vi "PhotonPoseEstimator_closestToCameraHeightStrategy.vi"(10 "CameraResult":T11, 11 "PhotonPoseEstimator_REF":T1) -> (1 "Pos Found":bool, 3 "PhotonEstimatedRobotPose":T2={"EstimatedPose"={"Translation3d"={"X"=0.0, "Y"=0.0, "Z"=0.0}, "Rotation3d"={"Q_quaternion"={"R"=1.0, "V"=[0.0, 0.0, 0.0]}}}, "TimeStamp_Seconds"=0.0, "targetsUsed"=[], "Strategy"=enum."LOWEST_AMBIGUITY"} {"targetsUsed"."AltCameraToTarget"."TRANSLATION3D"."Z" format="%14.3f"; "targetsUsed"."AltCameraToTarget"."TRANSLATION3D"."Y" format="%14.3f"; "targetsUsed"."AltCameraToTarget"."TRANSLATION3D"."X" format="%14.3f"; "targetsUsed"."BestCameraToTarget"."TRANSLATION3D"."Z" format="%14.3f"; "targetsUsed"."BestCameraToTarget"."TRANSLATION3D"."Y" format="%14.3f"; "targetsUsed"."BestCameraToTarget"."TRANSLATION3D"."X" format="%14.3f"; "EstimatedPose"."Translation3d"."Z" format="%14.3f"; "EstimatedPose"."Translation3d"."Y" format="%14.3f"; "EstimatedPose"."Translation3d"."X" format="%14.3f"})   [LabVIEW 2019, in "PhotonVisionLib.lvlib"]
doc: "This is an internal function. Use Update or Update_Pipeline instead of this function.\n\nDetermine the best target based on the target height closed to the camera height."
uses:
  PhotonVisionLib.lvlib
  <vilib>/Rock Robotics/WPI/ThirdParty/JAS_Junk/TrajLib/TypeDef/QUATERNION.ctl
  <vilib>/Rock Robotics/WPI/ThirdParty/JAS_Junk/TrajLib/Trajectory_Library.lvlib
  <vilib>/Rock Robotics/WPI/ThirdParty/JAS_Junk/TrajLib/TypeDef/ROTATION3D.ctl
  <vilib>/Rock Robotics/WPI/ThirdParty/JAS_Junk/TrajLib/TypeDef/TRANSLATION3D.ctl
  <vilib>/Rock Robotics/WPI/ThirdParty/JAS_Junk/TrajLib/TypeDef/POSE3D.ctl
  TypeDef/PhotonEstimatedRobotPoseType.ctl
  Enum/PhotonPoseStrategy_ENUM.ctl
  TypeDef/TargetCornerType.ctl
  <vilib>/Rock Robotics/WPI/ThirdParty/JAS_Junk/TrajLib/TypeDef/TRANSFORM3D.ctl
  TypeDef/PhotonTrackedTargetType.ctl
  TypeDef/PhotonPipelineResultType.ctl
  <vilib>/Rock Robotics/WPI/ThirdParty/JAS_Junk/TrajLib/TypeDef/AprilTag.ctl
  <vilib>/Rock Robotics/WPI/ThirdParty/JAS_Junk/TrajLib/Enum/AprilTagFieldLayoutOrignPosition_ENUM.ctl
  <vilib>/Rock Robotics/WPI/ThirdParty/JAS_Junk/TrajLib/TypeDef/AprilTagFieldLayout.ctl
  TypeDef/PhotonPoseEstimatorType.ctl
  TypeDef/PhotonPNPResultType.ctl
  TypeDef/PhotonMultiTargetPNPResultType.ctl
  TypeDef/PhotonTargetModel.ctl
  Ref/PhotonPipelineResult_REF.ctl
  Ref/PhotonPoseEstimator_REF.ctl
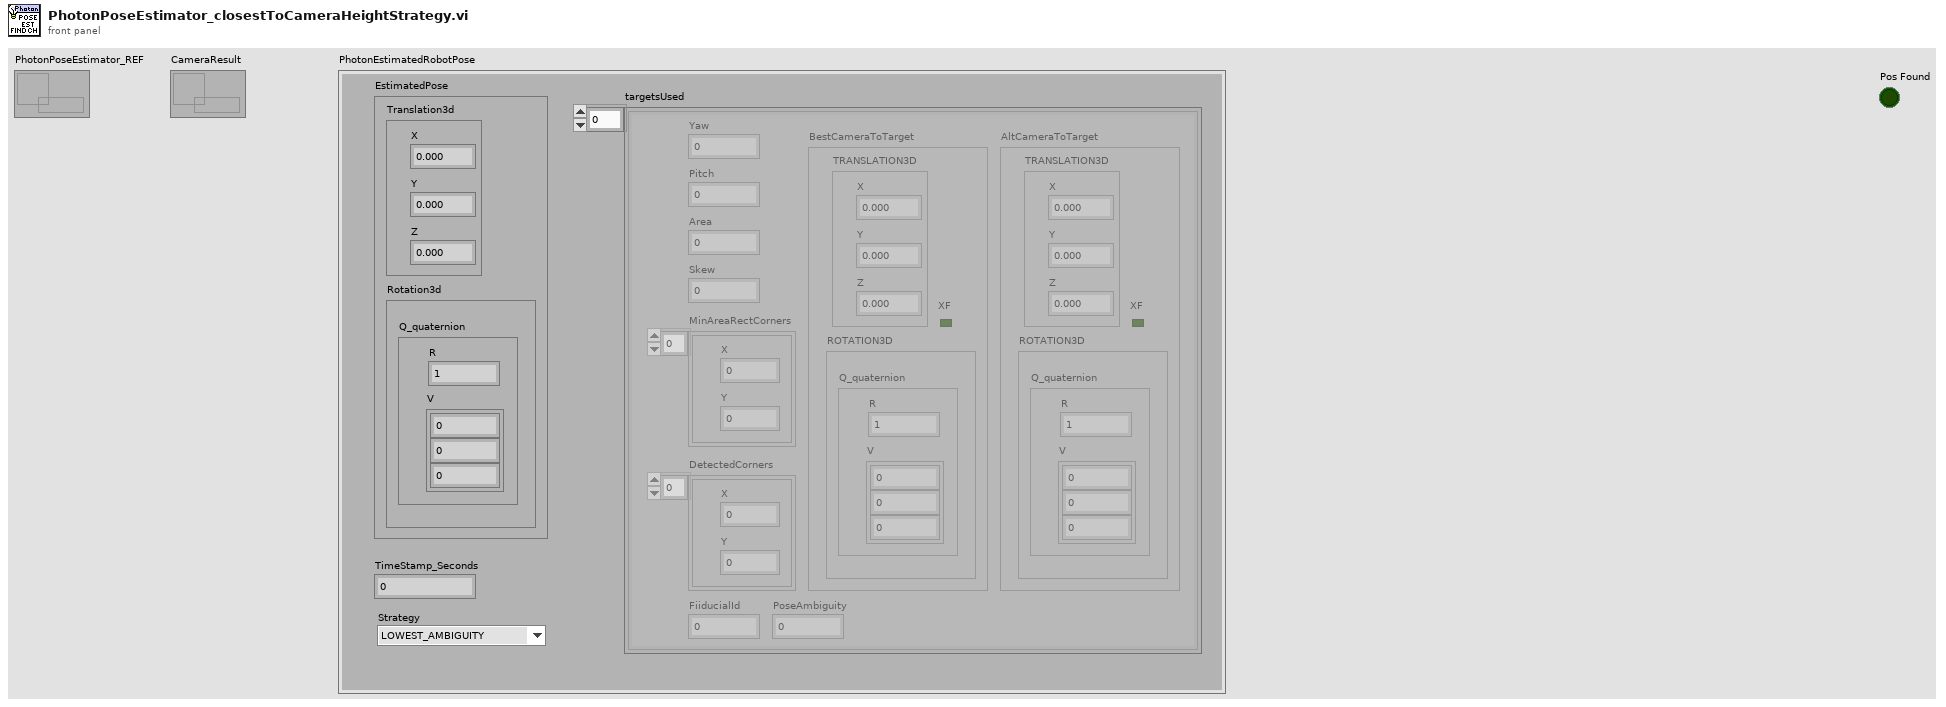
[diagram p1: front panel]
types:
  T1 = typedef "PhotonVisionLib.lvlib/PhotonPoseEstimator_REF.ctl" = refnum<data-value>
  T2 = typedef "PhotonVisionLib.lvlib/PhotonEstimatedRobotPoseType.ctl" = cluster{"EstimatedPose":T3, "TimeStamp_Seconds":dbl, "targetsUsed":T7[], "Strategy":T10}
  T3 = typedef "Trajectory_Library.lvlib/POSE3D.ctl" = cluster{"Translation3d":T4, "Rotation3d":T5}
  T4 = typedef "Trajectory_Library.lvlib/TRANSLATION3D.ctl" = cluster{"X":dbl, "Y":dbl, "Z":dbl}
  T5 = typedef "Trajectory_Library.lvlib/ROTATION3D.ctl" = cluster{"Q_quaternion":T6}
  T6 = typedef "Trajectory_Library.lvlib/QUATERNION.ctl" = cluster{"R":dbl, "V":dbl[]}
  T7 = typedef "PhotonVisionLib.lvlib/PhotonTrackedTargetType.ctl" = cluster{"Yaw":dbl, "Pitch":dbl, "Area":dbl, "Skew":dbl, "MinAreaRectCorners":T8[], "BestCameraToTarget":T9, "FiiducialId":i32, "AltCameraToTarget":T9, "PoseAmbiguity":dbl, "DetectedCorners":T8[]}
  T8 = typedef "PhotonVisionLib.lvlib/TargetCornerType.ctl" = cluster{"X":dbl, "Y":dbl}
  T9 = typedef "Trajectory_Library.lvlib/TRANSFORM3D.ctl" = cluster{"TRANSLATION3D":T4, "ROTATION3D":T5, "XF":bool}
  T10 = typedef "PhotonVisionLib.lvlib/PhotonPoseStrategy_ENUM.ctl" = enum16{"LOWEST_AMBIGUITY", "CLOSEST_TO_CAMERA_HEIGHT", "CLOSEST_TO_REFERENCE_POSE", "CLOSEST_TO_LAST_POSE", "AVERAGE_BEST_TARGETS", "MULTI_TAG_PNP_ON_COPROCESSOR", "MULTI_TAG_PNP_ON_RIO"}
  T11 = typedef "PhotonVisionLib.lvlib/PhotonPipelineResult_REF.ctl" = refnum<data-value>
  T12 = typedef "Trajectory_Library.lvlib/AprilTagFieldLayout.ctl" = cluster{"AprilTagMap":map{i32, T13}, "FieldLength":dbl, "FieldWidth":dbl, "OriginPosition ":T14, "OriginPose3d":T3}
  T13 = typedef "Trajectory_Library.lvlib/AprilTag.ctl" = cluster{"ID":i32, "POSE3D":T3}
  T14 = typedef "Trajectory_Library.lvlib/AprilTagFieldLayoutOrignPosition_ENUM.ctl" = enum16{"kBlueAllianceWallRightSide,", "kRedAllianceWallRightSide,"}
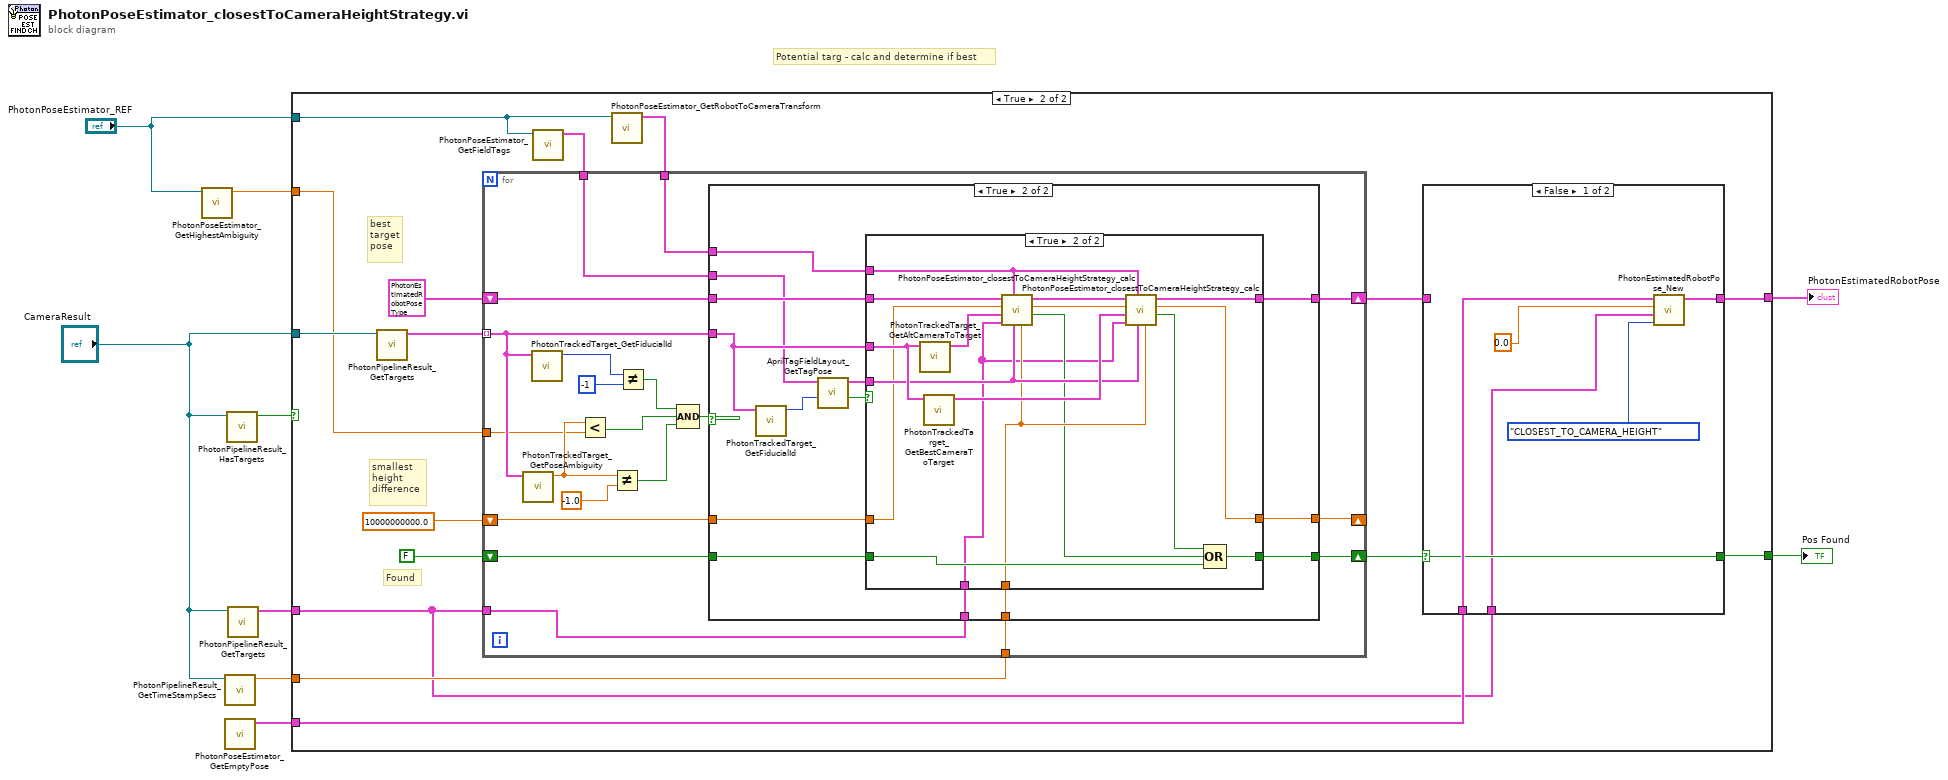
[diagram p0: block diagram]
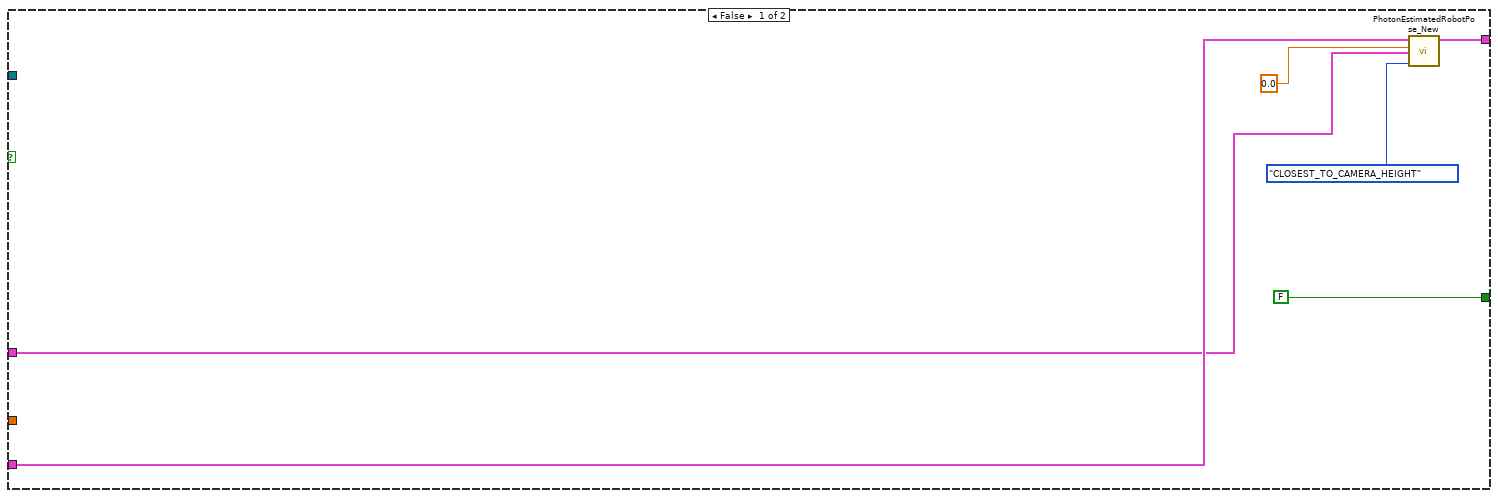
[diagram p2: hidden frame]
diagram:
  # "Potential targ - calc and determine if best"
  n1 = call "PhotonPoseEstimator_GetHighestAmbiguity.vi"("PhotonPoseEstimator"="PhotonPoseEstimator_REF") -> ("HighestAmbiguity"=w3:dbl)  [unwired: 10 in]
  n2 = call "PhotonPipelineResult_GetTimeStampSecs.vi"("PhotonPipelineResult_REF"="CameraResult") -> ("TimeStampSec"=w8:dbl)  [unwired: 10 in]
  n3 = call "PhotonPoseEstimator_GetEmptyPose.vi"() -> ("EmptyPose"=w7:T3)  [unwired: 11 in]
  n4 = call "PhotonPipelineResult_HasTargets.vi"("PhotonPipelineResult_REF"="CameraResult") -> ("HasTargets"=w9:bool)  [unwired: 10 in]
  n5 = call "PhotonPipelineResult_GetTargets.vi"("PhotonPipelineResult_REF"="CameraResult") -> ("Targets"=w1:T7[])  [unwired: 10 in]
  n6 = case shown="True" w9 {
    tunnel: "CameraResult" -> [_ w28]
    tunnel: [FALSE ("Found") w24] -> w5
    tunnel: "PhotonPoseEstimator_REF" -> [_ w19]
    tunnel: w8 -> [_ w26]
    tunnel: [w14 w22] -> w6
    tunnel: w7 -> [w13 w21]
    tunnel: w3 -> [_ w20]
    tunnel: w1 -> [w10 w16]
    frame False {
      n7 = call "PhotonEstimatedRobotPose_New.vi"("Strategy"=PhotonPoseStrategy_ENUM."CLOSEST_TO_CAMERA_HEIGHT", "targetsUsed"=w10, "TimeStamp_Seconds"=0.0, "EstimatedPose"=w13) -> ("PhotonEstimatedRobotPose"=w14:T2)  [unwired: 7 in]
    }
    frame True {
      # "smallest\nheight\ndifference"
      # "best \ntarget\npose"
      # "Found"
      n8 = call "PhotonPipelineResult_GetTargets.vi"("PhotonPipelineResult_REF"=w28) -> ("Targets"=w31:T7[])  [unwired: 10 in]
      n9 = call "PhotonPoseEstimator_GetFieldTags.vi"("PhotonPoseEstimator"=w19) -> ("AprilTagFieldLayout"=w18:T12)  [unwired: 10 in]
      n10 = call "PhotonPoseEstimator_GetRobotToCameraTransform.vi"("PhotonPoseEstimator"=w19) -> ("RobotToCamera"=w17:T9)  [unwired: 10 in]
      n11 = for {
        tunnel: w31 -> [w51] mode=indexing
        shift-right: [w55] -> w23
        shift-left: T2 {"EstimatedPose"={"Translation3d"={"X"=0.0, "Y"=0.0, "Z"=0.0}, "Rotation3d"={"Q_quaternion"={"R"=1.0, "V"=[0.0, 0.0, 0.0]}}}, "TimeStamp_Seconds"=0.0, "targetsUsed"=[], "Strategy"=enum."LOWEST_AMBIGUITY"} ("PhotonEstimatedRobotPose") -> [w54]
        shift-right: [w59] -> w25
        shift-left: FALSE -> [w56]
        shift-right: [w58] -> _
        shift-left: 10000000000.0 -> [w57]
        tunnel: w26 -> [w47]
        tunnel: w20 -> [w45]
        tunnel: w18 -> [w42]
        tunnel: w17 -> [w41]
        tunnel: w16 -> [w40]
        n12 = call "PhotonTrackedTarget_GetPoseAmbiguity.vi"("TrackedTarget"=w51) -> ("Pose Ambiguity"=w46:dbl)  [unwired: 10 in]
        n13 = call "PhotonTrackedTarget_GetFiducialId.vi"("TrackedTarget"=w51) -> ("Fiducial Id"=w53:i32)  [unwired: 10 in]
        n14 = Less?(x=w46, y=w45) -> (x < y?=w43:bool)
        n15 = Not Equal?(x=w46, y=-1.0) -> (x != y?=w49:bool)
        n16 = Not Equal?(x=w53, y=-1) -> (x != y?=w44:bool)
        n17 = Compound Arithmetic op=AND(w44, w43, w49) -> (w48:bool)
        n18 = case shown="True" w48 {
          tunnel: [w61 w69] -> w59
          tunnel: [w62 w75] -> w58
          tunnel: w57 -> [w62 w68]
          tunnel: w56 -> [w61 w67]
          tunnel: w51 -> [_ w73]
          tunnel: [w60 w74] -> w55
          tunnel: w54 -> [w60 w76]
          tunnel: w47 -> [_ w66]
          tunnel: w42 -> [_ w65]
          tunnel: w41 -> [_ w64]
          tunnel: w40 -> [_ w63]
          frame False {
          }
          frame True {
            n19 = call "PhotonTrackedTarget_GetFiducialId.vi"("TrackedTarget"=w73) -> ("Fiducial Id"=w72:i32)  [unwired: 10 in]
            n20 = call <vilib>:"AprilTagFieldLayout_GetTagPose.vi"("TagId"=w72, "AprilTagFieldLayout"=w65) -> ("Found"=w71:bool, "TagPose3d"=w70:T3)  [unwired: 8 in]
            n21 = case shown="True" w71 {
              tunnel: w76 -> [w79 w84]
              tunnel: [w78 w81] -> w75
              tunnel: [w79 w94] -> w74
              tunnel: w64 -> [_ w86]
              tunnel: w73 -> [_ w93]
              tunnel: w70 -> [_ w92]
              tunnel: [w77 w91] -> w69
              tunnel: w68 -> [w78 w83]
              tunnel: w67 -> [w77 w90]
              tunnel: w66 -> [_ w89]
              tunnel: w63 -> [_ w80]
              frame False {
              }
              frame True {
                n22 = call "PhotonTrackedTarget_GetAltCameraToTarget.vi"("TrackedTarget"=w93) -> ("AltCameraToTarget"=w95:T9)  [unwired: 9 in, 1 out]
                n23 = call "PhotonTrackedTarget_GetBestCameraToTarget.vi"("TrackedTarget"=w93) -> ("BestCameraToTarget"=w96:T9)  [unwired: 9 in, 1 out]
                n24 = call "PhotonPoseEstimator_closestToCameraHeightStrategy_calc.vi"("TimeStamp"=w89, "FieldTargetPose"=w92, "RobotToCam"=w86, "Targets"=w80, "TransformToEvaluate"=w95, "SmallestHeightDiff"=w83, "CurrentBestTrackedTarg"=w84) -> ("Found New Best"=w87:bool, "SmallestHieghtDiff"=w82:dbl, "PhotonEstimatedRobotPose"=w85:T2)  [unwired: 2 in]
                n25 = call "PhotonPoseEstimator_closestToCameraHeightStrategy_calc.vi"("TimeStamp"=w89, "FieldTargetPose"=w92, "RobotToCam"=w86, "Targets"=w80, "TransformToEvaluate"=w96, "SmallestHeightDiff"=w82, "CurrentBestTrackedTarg"=w85) -> ("Found New Best"=w88:bool, "SmallestHieghtDiff"=w81:dbl, "PhotonEstimatedRobotPose"=w94:T2)  [unwired: 2 in]
                n26 = Compound Arithmetic op=OR(w88, w87, w90) -> (w91:bool)
              }
            }
          }
        }
      }
      n27 = case shown="False" w25 {
        selector: w25 -> [w35 w39]
        tunnel: [w35 w39] -> w24
        tunnel: [w36 w38] -> w22
        tunnel: w23 -> [_ w38]
        tunnel: w21 -> [w37 _]
        tunnel: w16 -> [w32 _]
        frame False {
          n28 = call "PhotonEstimatedRobotPose_New.vi"("Strategy"=PhotonPoseStrategy_ENUM."CLOSEST_TO_CAMERA_HEIGHT", "targetsUsed"=w32, "TimeStamp_Seconds"=0.0, "EstimatedPose"=w37) -> ("PhotonEstimatedRobotPose"=w36:T2)  [unwired: 7 in]
        }
        frame True {
        }
      }
    }
  }
  "PhotonEstimatedRobotPose" <- w6
  "Pos Found" <- w5
